vi "Log Parse.vi"(7 "offset (in bytes) (1000000)":i64=1000000, 9 "Duration":dbl=30.0, 10 "CSV Refnum Files":path[](array[path]), 11 "OEM 719 Simulated Log":path) -> (1 "Elapsed_time":dbl format="%<%H:%M:%S%2u>t", 8 "error out":errorcluster)   [LabVIEW 2025]
panel:
  out "Final Output":string[](array[string])
  out "text":string[](array[string])
  out "Offset":i32
  in  "error in":errorcluster
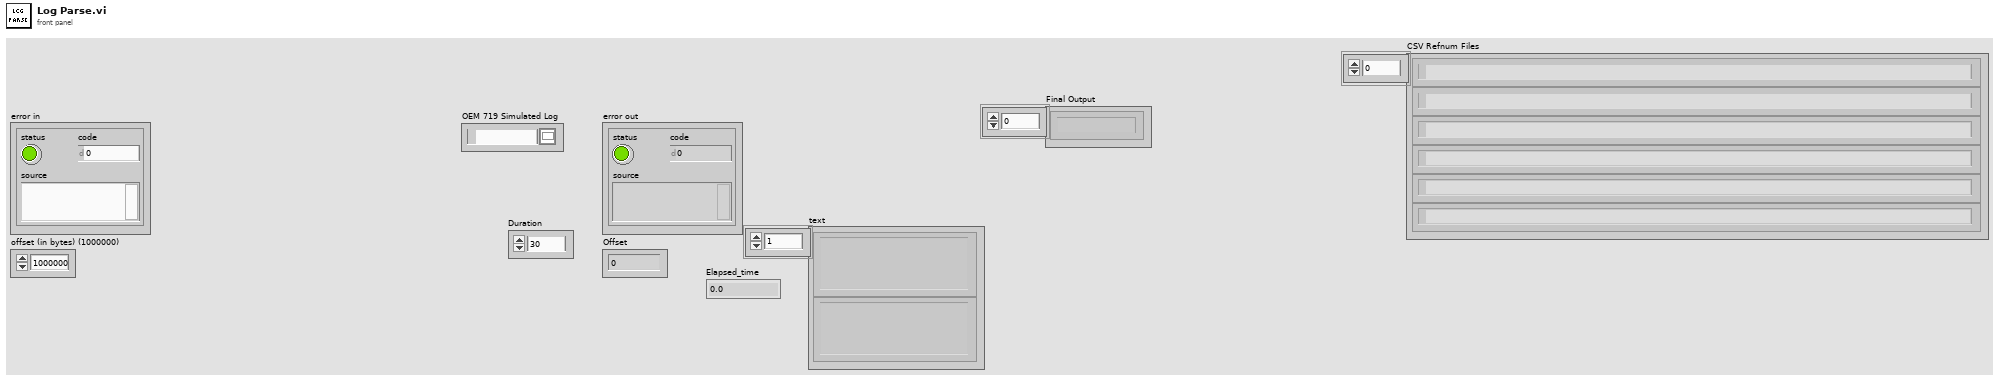
[diagram p1: front panel]
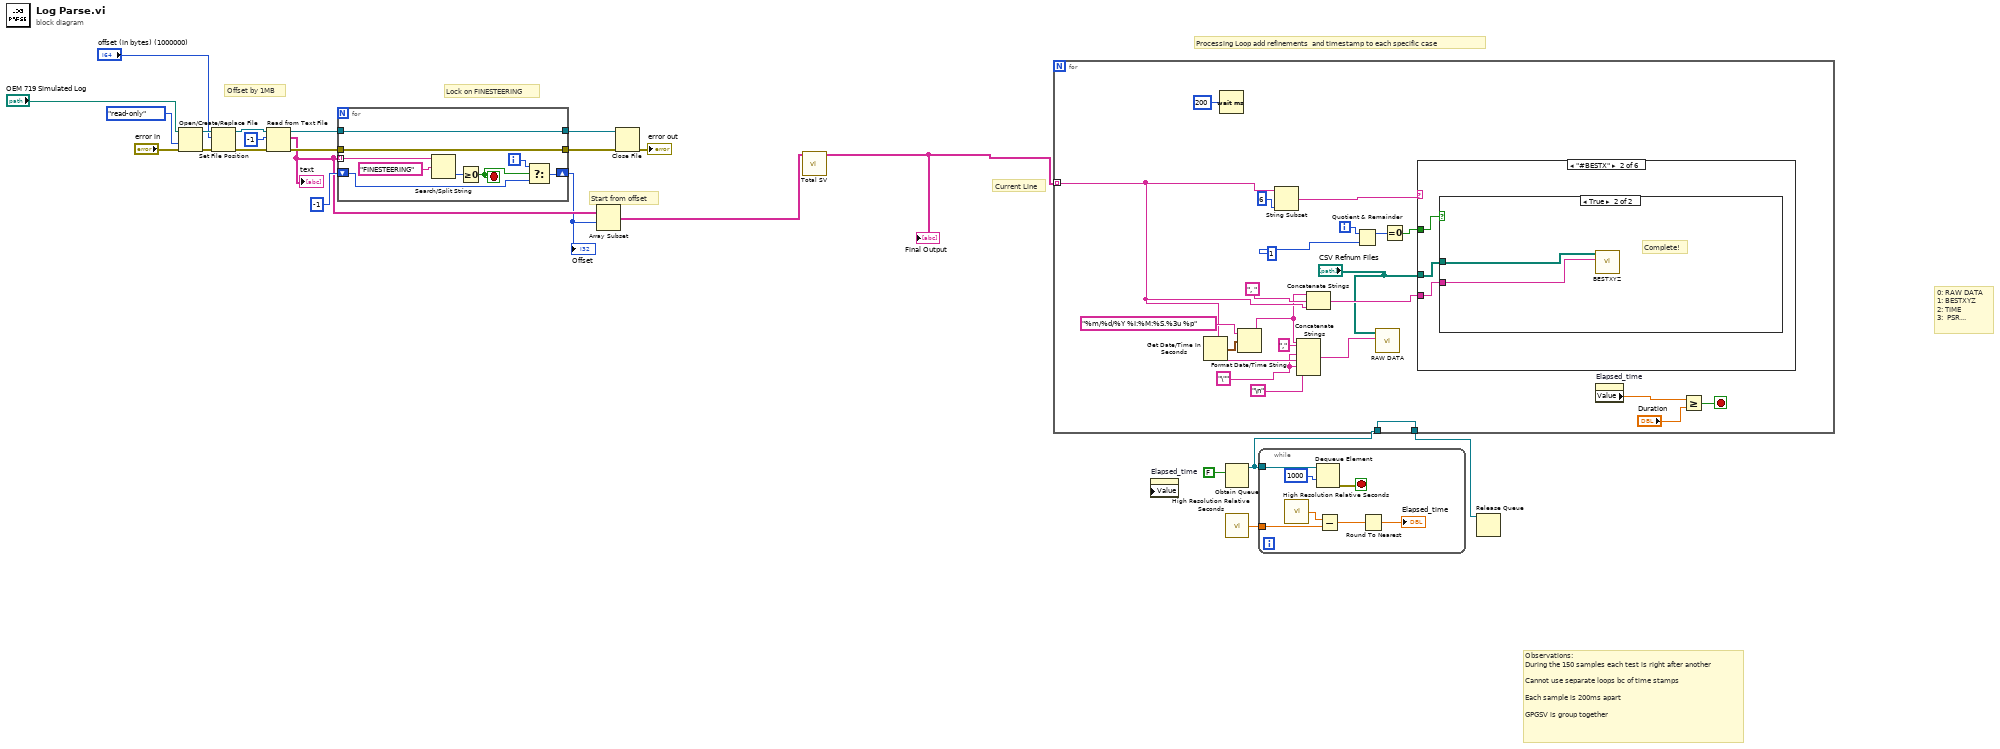
[diagram p0: block diagram]
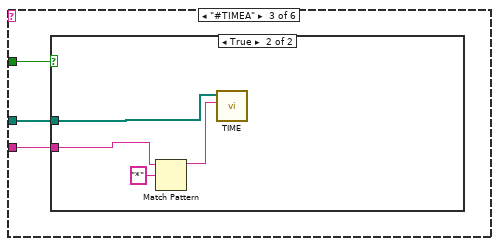
[diagram p4: hidden frame]
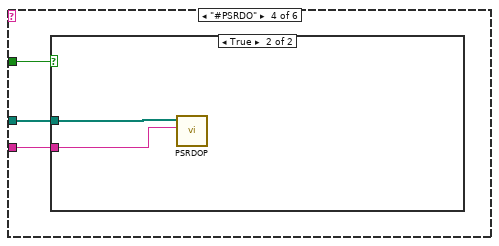
[diagram p6: hidden frame]
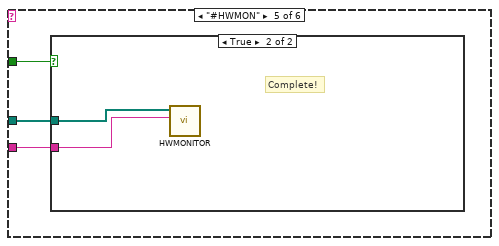
[diagram p8: hidden frame]
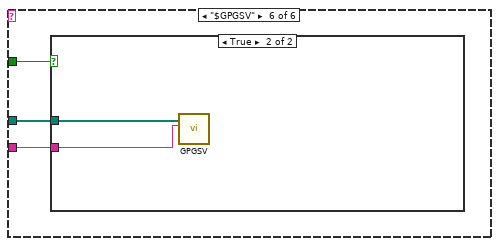
[diagram p10: hidden frame]
diagram:
  # "Start from offset"
  # "Lock on FINESTEERING"
  # "Offset by 1MB"
  # "Observations:\nDuring the 150 samples each test is right after another\n\nCannot use separate loops bc of time stamps\n\nEach sample is 200ms apart\n\nGPGSV is group together"
  # "0: RAW DATA\n1: BESTXYZ\n2: TIME\n3:  PSR..."
  # "Current Line"
  # "Processing Loop add refinements  and timestamp to each specific case"
  n1 = Open/Create/Replace File(file path (use dialog)="OEM 719 Simulated Log", error in="error in", access (0:read/write)=enum16{"read/write", "read-only", "write-only"}."read-only") -> (refnum out=w22:refnum<file>, error out=w14:errorcluster)  [unwired: 3 in, 1 out]
  n2 = Set File Position(offset (in bytes) (0)="offset (in bytes) (1000000)", refnum=w22, error in=w14) -> (refnum out=w21:refnum<file>, error out=w13:errorcluster)  [unwired: 1 in]
  n3 = Read from Text File(file (use dialog)=w21, count=-1, error in=w13) -> (refnum out=w17:refnum<file>, text=w9:string[], error out=w12:errorcluster)  [unwired: 1 in, 1 out]
  "text" <- w9
  n4 = for {
    tunnel: w9 -> [w32] mode=indexing
    shift-right: [w27] -> w8
    shift-left: -1 -> [w28]
    tunnel: w17 -> [w25]
    tunnel: [w25] -> w16
    tunnel: w12 -> [w24]
    tunnel: [w24] -> w11
    i -> [w29]
    stop <- w26 stop-if-true
    n5 = Search/Split String(string=w32, search string/char (-)="FINESTEERING" ("regular expression")) -> (offset of match=w30:i32)  [unwired: 1 in, 2 out]
    n6 = Greater Or Equal To 0?(x=w30) -> (x >= 0?=w26:bool)
    n7 = Select(t=w29, s=w26, f=w28) -> (s? t:f=w27:i32)
  }
  "Offset" <- w8
  n8 = Array Subset(array=w9, index=w8) -> (w2:string[])  [unwired: 1 in]
  n9 = Close File(refnum=w16, error in=w11) -> (error out=→"error out":errorcluster)  [unwired: 1 out]
  n10 = call "Total SV.vi"("All Lines"=w2) -> ("Final Output"=w1:string[])  [unwired: 10 in]
  "Final Output" <- w1
  n11 = property on="Elapsed_time" class="DigNum (strict)" props=["Value"]() -> ()  [unwired: 3 in, 2 out]
  n12 = Obtain Queue(element data type=FALSE) -> (queue out=w4:refnum<queue>)  [unwired: 4 in, 2 out]
  n13 = for {
    tunnel: w1 -> [w39] mode=indexing
    tunnel: w4 -> [w52]
    tunnel: [w52] -> w3
    i -> [w48]
    stop <- w51 stop-if-true
    w34 = "\""
    n14 = Get Date/Time In Seconds() -> (seconds since 1Jan1904=w46:timestamp)
    n15 = Wait (ms)(milliseconds to wait=u32 200) -> ()  [unwired: 1 out]
    n16 = Format Date/Time String(time format string (%c)="%m/%d/%Y %I:%M:%S.%3u %p", seconds (now)=w46) -> (date/time string=w38:string)  [unwired: 1 in]
    n17 = String Subset(string=w39, length (rest)=6 ("length (rest)")) -> (substring=w43:string)  [unwired: 1 in]
    n18 = Concatenate Strings(w38, "," ("string"), w34, w39, w34, "\n") -> (w37:string)
    n19 = Concatenate Strings(w38, ", " ("string"), w39) -> (w42:string)
    n20 = Quotient & Remainder(x=w48, y=1) -> (x-y*floor(x/y)=w47:i32)  [unwired: 1 out]
    n21 = call "RAW DATA.vi"("String"=w37, "array"="CSV Refnum Files") -> ()  [unwired: 9 in, 1 out]
    n22 = Equal To 0?(x=w47) -> (x = 0?=w44:bool)
    n23 = case shown="\"#BESTX\"" w43 {
      tunnel: w44 -> [_ w57 w62 w69 w74 w79]
      tunnel: "CSV Refnum Files" -> [_ w56 w61 w68 w73 w78]
      tunnel: w42 -> [_ w55 w60 w67 w72 w77]
      frame "RAW DATA", Default {
      }
      frame "#BESTX" {
        n24 = case shown="True" w57 {
          tunnel: w56 -> [_ w59]
          tunnel: w55 -> [_ w58]
          frame False {
            # "Raw Data"
          }
          frame True {
            # "Complete!"
            n25 = call "BESTXYZ.vi"("String"=w58, "array"=w59) -> ()  [unwired: 9 in, 1 out]
          }
        }
      }
      frame "#TIMEA" {
        n26 = case shown="True" w62 {
          tunnel: w61 -> [_ w66]
          tunnel: w60 -> [_ w64]
          frame False {
            # "Raw Data"
          }
          frame True {
            n27 = Match Pattern(string=w64, regular expression="*") -> (before substring=w63:string)  [unwired: 1 in, 3 out]
            n28 = call "TIME.vi"("String"=w63, "array"=w66) -> ()  [unwired: 9 in, 1 out]
          }
        }
      }
      frame "#PSRDO" {
        n29 = case shown="True" w69 {
          tunnel: w68 -> [_ w71]
          tunnel: w67 -> [_ w70]
          frame False {
            # "Raw Data"
          }
          frame True {
            n30 = call "PSRDOP.vi"("String"=w70, "array"=w71) -> ()  [unwired: 9 in, 1 out]
          }
        }
      }
      frame "#HWMON" {
        n31 = case shown="True" w74 {
          tunnel: w73 -> [_ w76]
          tunnel: w72 -> [_ w75]
          frame False {
            # "Raw Data"
          }
          frame True {
            # "Complete!"
            n32 = call "HWMONITOR.vi"("String"=w75, "array"=w76) -> ()  [unwired: 9 in, 1 out]
          }
        }
      }
      frame "$GPGSV" {
        n33 = case shown="True" w79 {
          tunnel: w78 -> [_ w81]
          tunnel: w77 -> [_ w80]
          frame False {
            # "Raw Data"
          }
          frame True {
            n34 = call "GPGSV.vi"("String"=w80, "array"=w81) -> ()  [unwired: 10 in]
          }
        }
      }
    }
    n35 = property on="Elapsed_time" class="DigNum (strict)"() -> ("Value"=w49:dbl)  [unwired: 2 in, 2 out]
    n36 = Greater Or Equal?(x=w49, y="Duration") -> (x >= y?=w51:bool)
  }
  n37 = call <vilib>:"High Resolution Relative Seconds.vi"() -> ("relative seconds"=w6:dbl)
  n38 = while {
    tunnel: w6 -> [w86]
    tunnel: w4 -> [w85]
    stop <- w83 stop-if-true
    n39 = call <vilib>:"High Resolution Relative Seconds.vi"() -> ("relative seconds"=w87:dbl)
    n40 = Dequeue Element(queue=w85, timeout in ms (-1)=1000) -> (error out=w83:errorcluster)  [unwired: 1 in, 3 out]
    n41 = Subtract(x=w87, y=w86) -> (x-y=w88:dbl)
    n42 = Round To Nearest(number=w88) -> (nearest integer value=→"Elapsed_time":dbl)
  }
  n43 = Release Queue(queue=w3) -> ()  [unwired: 2 in, 3 out]
